vi "serial_clear_reset_wait.vi"(0 "VISA Refnum in":refnum<visa-resource-name>, 1 "error in (no error)":errorcluster) -> (2 "VISA Refnum out":refnum<visa-resource-name>, 3 "test":bool, 4 "error out":errorcluster)   [LabVIEW 2019]
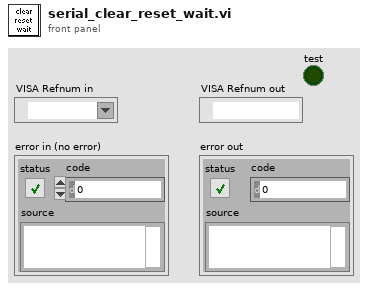
[diagram p1: front panel]
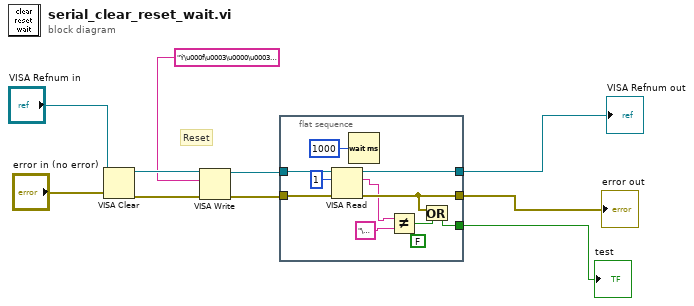
[diagram p0: block diagram]
diagram:
  # "Reset"
  n1 = VISA Clear(VISA resource name="VISA Refnum in", error in (no error)="error in (no error)") -> (VISA resource name out=w5:refnum<visa-resource-name>, error out=w6:errorcluster)
  n2 = VISA Write(VISA resource name=w5, write buffer="Ý\u000f\u0003\u0000\u0003\u0000w", error in (no error)=w6) -> (VISA resource name out=w9:refnum<visa-resource-name>, error out=w10:errorcluster)  [unwired: 1 out]
  n3 = flat-sequence {
    tunnel: [w17] -> w7
    tunnel: w9 -> [w19]
    tunnel: w10 -> [w18]
    tunnel: [w15] -> w8
    tunnel: [w12] -> w1
    frame #0 {
      (unwired) FALSE
      n4 = VISA Read(VISA resource name=w19, byte count=u32 1, error in (no error)=w18) -> (VISA resource name out=w17:refnum<visa-resource-name>, read buffer=w14:string, error out=w15:errorcluster)  [unwired: 1 out]
      n5 = Wait (ms)(milliseconds to wait=u32 1000) -> ()  [unwired: 1 out]
      n6 = Not Equal?(x=w14, y="\u0001") -> (x != y?=w11:bool)
      n7 = Or(x=w15, y=w11) -> (x .or. y?=w12:bool)
    }
  }
  "error out" <- w8
  "VISA Refnum out" <- w7
  "test" <- w1
